vi "ChannelSettings2.vi"(8 "error in (no error)":errorcluster, 9 "ChannelCluster":T1 {"Range" items=["0.2 Vpp"=0.2, "0.4 Vpp"=0.4, "0.8 Vpp"=0.8, "2 Vpp"=2.0, "4 Vpp"=4.0, "8 Vpp"=8.0, "20 Vpp"=20.0, "80 Vpp"=80.0]}, 10 "NChans":i32, 11 "hDevice in":u32) -> (0 "error out":errorcluster, 3 "hDevice out":u32)   [LabVIEW 2018]
uses:
  LibTiePie.lvlib
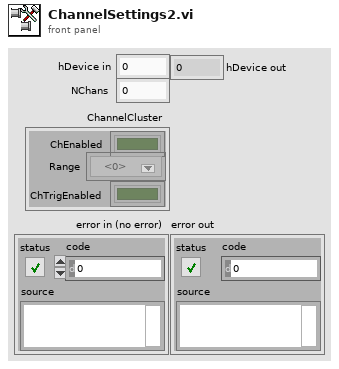
[diagram p1: front panel]
types:
  T1 = cluster{"ChEnabled":bool[], "Range":dbl[], "ChTrigEnabled":bool[]}
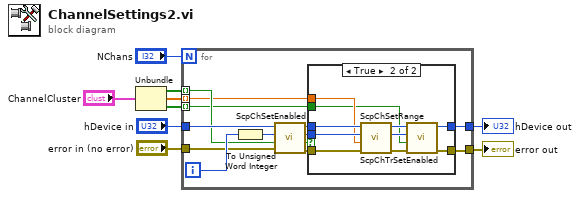
[diagram p0: block diagram]
diagram:
  n1 = Unbundle("ChannelCluster") -> ("ChEnabled"=w5:bool[], "Range"=w4:dbl[], "ChTrigEnabled"=w3:bool[])
  n2 = for {
    N: "NChans" -> [_]
    tunnel: "hDevice in" -> [w19]
    tunnel: "error in (no error)" -> [w16]
    tunnel: [w15] -> w2
    tunnel: [w14] -> w1
    tunnel: w5 -> [w12] mode=indexing
    tunnel: w4 -> [w11] mode=indexing
    tunnel: w3 -> [w10] mode=indexing
    i -> [w18]
    n3 = To Unsigned Word Integer(number=w18) -> (unsigned 16bit integer=w17:u16)
    n4 = call "ScpChSetEnabled.vi"("error in (no error)"=w16, "Enable?"=w12, "wCh in"=w17, "hDevice in"=w19) -> ("error out"=w21:errorcluster, "Enabled?"=w13:bool, "wCh out"=w20:u16, "hDevice out"=w22:u32)  [unwired: 4 in]
    n5 = case shown="True" w13 {
      tunnel: w22 -> [w24 w34]
      tunnel: w21 -> [w23 w32]
      tunnel: w20 -> [_ w30]
      tunnel: [w23 w28] -> w15
      tunnel: [w24 w27] -> w14
      tunnel: w11 -> [_ w26]
      tunnel: w10 -> [_ w25]
      frame False {
      }
      frame True {
        n6 = call "ScpChSetRange.vi"("error in (no error)"=w32, "dRange"=w26, "wCh"=w30, "hDevice in"=w34) -> ("error out"=w31:errorcluster, "wCh out"=w29:u16, "hDevice out"=w33:u32)  [unwired: 4 in, 1 out]
        n7 = call "ScpChTrSetEnabled.vi"("error in (no error)"=w31, "TrigEnable"=w25, "wCh"=w29, "hDevice"=w33) -> ("error out"=w28:errorcluster, "hDevice out"=w27:u32)  [unwired: 4 in, 2 out]
      }
    }
  }
  "error out" <- w2
  "hDevice out" <- w1
